vi "Test Assert Duplicate AssertName.vi"(8 "error in (no error)":errorcluster) -> (0 "error out":errorcluster)   [LabVIEW 2013]
uses:
  classes/Test/Test.lvclass
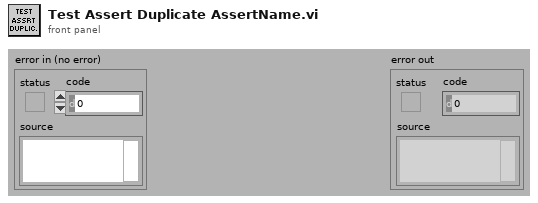
[diagram p1: front panel]
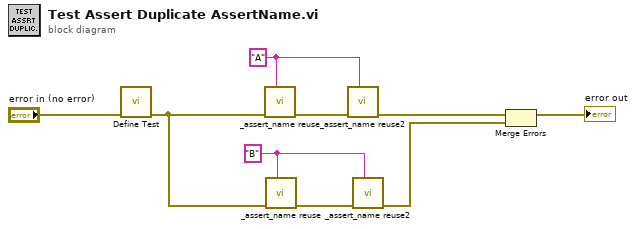
[diagram p0: block diagram]
diagram:
  w3 = "B" ("Name")
  w4 = "A" ("Name")
  n1 = call "Define Test.vi"("error in (no error)"="error in (no error)") -> ("error out"=w1:errorcluster)  [unwired: 10 in]
  n2 = call "_assert_name reuse.vi"("Name"=w4, "error in (no error)"=w1) -> ("error out"=w6:errorcluster)  [unwired: 9 in]
  n3 = call "_assert_name reuse.vi"("Name"=w3, "error in (no error)"=w1) -> ("error out"=w2:errorcluster)  [unwired: 9 in]
  n4 = call "_assert_name reuse2.vi"("Name"=w4, "error in (no error)"=w6) -> ("error out"=w5:errorcluster)  [unwired: 9 in]
  n5 = call "_assert_name reuse2.vi"("Name"=w3, "error in (no error)"=w2) -> ("error out"=w7:errorcluster)  [unwired: 9 in]
  n6 = Merge Errors(w5, w7) -> (→"error out":errorcluster)
